vi "Lab Panel V5.28.vi"() -> ()   [LabVIEW 2013] (continued)
              tunnel: w5214 -> [_ w5263]
              tunnel: w5224 -> [_ w5262]
              tunnel: w5223 -> [_ w5261]
              tunnel: w5222 -> [_ w5260]
              tunnel: w5221 -> [_ w5259]
              tunnel: w5220 -> [_ w5258]
              tunnel: w5219 -> [_ w5257]
              tunnel: w5218 -> [_ w5256]
              tunnel: w5217 -> [_ w5255]
              tunnel: w5216 -> [_ w5254]
              tunnel: w5215 -> [_ w5253]
              tunnel: "TO (string):" -> [w5229 _]
              frame #0 {
                # "mail test"
                n2896 = case shown="True" w5230 {
                  tunnel: w5233 -> [_ w5237]
                  tunnel: w5229 -> [_ w5236]
                  tunnel: w5232 -> [_ w5235]
                  tunnel: w5231 -> [_ w5234]
                  frame False {
                  }
                  frame True {
                    n2897 = stacked-sequence {
                      seq-local: [_ _ w5247 _] -> [_ _ _ w5248]
                      tunnel: w5237 -> [w5240 _ _ w5252]
                      tunnel: w5236 -> [_ _ w5245 _]
                      tunnel: w5235 -> [_ _ w5243 _]
                      tunnel: w5234 -> [_ _ w5244 _]
                      frame #0 {
                        n2898 = Bundle(cluster=w5240, "TEST MAIL STATUS"="TEST START") -> (w5238:T7)  [unwired: 6 in]
                        n2899 = local write "MAIL SETTINGS"(w5238) -> ()
                      }
                      frame #1 {
                        n2900 = Wait (ms)(milliseconds to wait=500) -> ()  [unwired: 1 out]
                      }
                      frame #2 {
                        n2901 = call "sub vi - send mail v5.vi"("TO:"=w5245, "subject"="MAIL TEST FROM LAB PANEL", "from"=w5244, "out going server"=w5243, "message"="TEST MESSAGE") -> ("error out"=w5247:errorcluster)  [unwired: 10 in]
                      }
                      frame #3 {
                        n2902 = Bundle(cluster=w5252, "TEST MAIL"=FALSE, "TEST MAIL STATUS"="TEST END", "mail error"=w5248) -> (w5250:T7)  [unwired: 4 in]
                        n2903 = local write "MAIL SETTINGS"(w5250) -> ()
                      }
                    }
                  }
                }
              }
              frame #1 {
                # "mail report"
                n2904 = stacked-sequence {
                  seq-local: [_ w5310 _ _] -> [_ _ _ w5500]
                  seq-local: [_ _ w5413 _] -> [_ _ _ w5490]
                  seq-local: [w5277 _ _ _] -> [_ w5327 _ _]
                  seq-local: [w5276 _ _ _] -> [_ w5326 _ _]
                  seq-local: [w5274 _ _ _] -> [_ w5324 _ _]
                  seq-local: [w5275 _ _ _] -> [_ w5325 _ _]
                  seq-local: [w5273 _ _ _] -> [_ w5323 _ _]
                  seq-local: [w5272 _ _ _] -> [_ w5318 _ _]
                  seq-local: [w5271 _ _ _] -> [_ w5319 _ _]
                  seq-local: [w5270 _ _ _] -> [_ w5320 _ _]
                  seq-local: [w5269 _ _ _] -> [_ w5321 _ _]
                  seq-local: [w5268 _ _ _] -> [_ w5322 _ _]
                  tunnel: w5267 -> [_ _ _ w5501]
                  tunnel: w5266 -> [_ _ _ w5484]
                  tunnel: w5265 -> [_ _ _ w5498]
                  tunnel: w5264 -> [_ _ _ w5497]
                  tunnel: w5263 -> [w5308 _ _ w5492]
                  tunnel: w5262 -> [_ _ w5443 _]
                  tunnel: w5261 -> [_ _ w5440 _]
                  tunnel: w5260 -> [_ _ w5439 _]
                  tunnel: w5259 -> [_ _ w5438 _]
                  tunnel: w5258 -> [_ _ w5437 _]
                  tunnel: w5257 -> [_ _ w5436 _]
                  tunnel: w5256 -> [_ _ w5435 _]
                  tunnel: w5255 -> [_ _ w5434 _]
                  tunnel: w5254 -> [_ _ w5433 _]
                  tunnel: w5253 -> [_ _ w5432 _]
                  frame #0 {
                    n2905 = case shown="False" w5308 {
                      frame False {
                        n2906 = local write "mail control"("") -> ()
                      }
                      frame True {
                      }
                    }
                    n2907 = local read "SET LAB01-1"() -> (w5307:T5)
                    n2908 = local read "SET LAB01-2"() -> (w5306:T5)
                    n2909 = local read "SET LAB02-1"() -> (w5305:T5)
                    n2910 = local read "SET LAB02-2"() -> (w5304:T5)
                    n2911 = local read "SET LAB03-1"() -> (w5303:T5)
                    n2912 = local read "SET LAB04-1"() -> (w5301:T5)
                    n2913 = local read "SET LAB05-1"() -> (w5299:T5)
                    n2914 = local read "SET LAB03-2"() -> (w5302:T5)
                    n2915 = local read "SET LAB04-2"() -> (w5300:T5)
                    n2916 = local read "SET LAB05-2"() -> (w5298:T5)
                    n2917 = Unbundle(w5303) -> ("DESCRIPTION"=w5283:string)  [unwired: 4 out]
                    n2918 = Unbundle(w5302) -> ("DESCRIPTION"=w5282:string)  [unwired: 4 out]
                    n2919 = Unbundle(w5301) -> ("DESCRIPTION"=w5281:string)  [unwired: 4 out]
                    n2920 = Unbundle(w5298) -> ("DESCRIPTION"=w5278:string)  [unwired: 4 out]
                    n2921 = Unbundle(w5304) -> ("DESCRIPTION"=w5284:string)  [unwired: 4 out]
                    n2922 = Unbundle(w5300) -> ("DESCRIPTION"=w5280:string)  [unwired: 4 out]
                    n2923 = Unbundle(w5307) -> ("DESCRIPTION"=w5296:string)  [unwired: 4 out]
                    n2924 = Unbundle(w5305) -> ("DESCRIPTION"=w5285:string)  [unwired: 4 out]
                    n2925 = Unbundle(w5299) -> ("DESCRIPTION"=w5279:string)  [unwired: 4 out]
                    n2926 = Unbundle(w5306) -> ("DESCRIPTION"=w5286:string)  [unwired: 4 out]
                    n2927 = Concatenate Strings("[LAB05-2/", w5278) -> (w5268:string)
                    n2928 = Concatenate Strings("[LAB05-1/", w5279) -> (w5269:string)
                    n2929 = Concatenate Strings("[LAB04-2/", w5280) -> (w5270:string)
                    n2930 = Concatenate Strings("[LAB03-2/", w5282) -> (w5272:string)
                    n2931 = Concatenate Strings("[LAB04-1/", w5281) -> (w5271:string)
                    n2932 = Concatenate Strings("[LAB03-1/", w5283) -> (w5273:string)
                    n2933 = Concatenate Strings("[LAB01-2/", w5286) -> (w5276:string)
                    n2934 = Concatenate Strings("[LAB02-2/", w5284) -> (w5274:string)
                    n2935 = Concatenate Strings("[LAB01-1/", w5296) -> (w5277:string)
                    n2936 = Concatenate Strings("[LAB02-1/", w5285) -> (w5275:string)
                  }
                  frame #1 {
                    w5331 = "/"
                    w5332 = 2.0
                    n2937 = local read "DISP LAB01-2"() -> (w5411:T4)
                    n2938 = local read "DISP LAB01-1"() -> (w5412:T4)
                    n2939 = local read "DISP LAB02-1"() -> (w5410:T4)
                    n2940 = local read "DISP LAB03-2"() -> (w5407:T4)
                    n2941 = local read "DISP LAB02-2"() -> (w5409:T4)
                    n2942 = local read "DISP LAB03-1"() -> (w5408:T4)
                    n2943 = local read "DISP LAB04-2"() -> (w5405:T4)
                    n2944 = local read "DISP LAB04-1"() -> (w5406:T4)
                    n2945 = local read "DISP LAB05-1"() -> (w5404:T4)
                    n2946 = local read "DISP LAB05-2"() -> (w5403:T4)
                    n2947 = Unbundle(w5411) -> ("CYCLE"=w5395:dbl, "MINS"=w5394:dbl, "STATUS"=w5391:string)
                    n2948 = Unbundle(w5412) -> ("CYCLE"=w5400:dbl, "MINS"=w5399:dbl, "STATUS"=w5396:string)
                    n2949 = Unbundle(w5410) -> ("CYCLE"=w5388:dbl, "MINS"=w5387:dbl, "STATUS"=w5386:string)
                    n2950 = Unbundle(w5407) -> ("CYCLE"=w5375:dbl, "MINS"=w5374:dbl, "STATUS"=w5371:string)
                    n2951 = Unbundle(w5408) -> ("CYCLE"=w5380:dbl, "MINS"=w5379:dbl, "STATUS"=w5376:string)
                    n2952 = Unbundle(w5409) -> ("CYCLE"=w5385:dbl, "MINS"=w5384:dbl, "STATUS"=w5381:string)
                    n2953 = Unbundle(w5406) -> ("CYCLE"=w5370:dbl, "MINS"=w5369:dbl, "STATUS"=w5366:string)
                    n2954 = Unbundle(w5405) -> ("CYCLE"=w5365:dbl, "MINS"=w5364:dbl, "STATUS"=w5361:string)
                    n2955 = Unbundle(w5404) -> ("CYCLE"=w5360:dbl, "MINS"=w5359:dbl, "STATUS"=w5356:string)
                    n2956 = Unbundle(w5403) -> ("CYCLE"=w5402:dbl, "MINS"=w5401:dbl, "STATUS"=w5353:string)
                    n2957 = Number To Decimal String(number=w5388) -> (decimal integer string=w5390:string)  [unwired: 1 in]
                    n2958 = Number To Decimal String(number=w5385) -> (decimal integer string=w5383:string)  [unwired: 1 in]
                    n2959 = Number To Decimal String(number=w5380) -> (decimal integer string=w5378:string)  [unwired: 1 in]
                    n2960 = Number To Decimal String(number=w5395) -> (decimal integer string=w5393:string)  [unwired: 1 in]
                    n2961 = Number To Decimal String(number=w5375) -> (decimal integer string=w5373:string)  [unwired: 1 in]
                    n2962 = Number To Decimal String(number=w5400) -> (decimal integer string=w5398:string)  [unwired: 1 in]
                    n2963 = Number To Decimal String(number=w5402) -> (decimal integer string=w5355:string)  [unwired: 1 in]
                    n2964 = Number To Decimal String(number=w5370) -> (decimal integer string=w5368:string)  [unwired: 1 in]
                    n2965 = Number To Decimal String(number=w5365) -> (decimal integer string=w5363:string)  [unwired: 1 in]
                    n2966 = Number To Decimal String(number=w5360) -> (decimal integer string=w5358:string)  [unwired: 1 in]
                    n2967 = Number To Fractional String(number=w5387, precision (6)=w5332) -> (F-format string=w5389:string)  [unwired: 2 in]
                    n2968 = Number To Fractional String(number=w5374, precision (6)=w5332) -> (F-format string=w5372:string)  [unwired: 2 in]
                    n2969 = Number To Fractional String(number=w5384, precision (6)=w5332) -> (F-format string=w5382:string)  [unwired: 2 in]
                    n2970 = Number To Fractional String(number=w5379, precision (6)=w5332) -> (F-format string=w5377:string)  [unwired: 2 in]
                    n2971 = Number To Fractional String(number=w5364, precision (6)=w5332) -> (F-format string=w5362:string)  [unwired: 2 in]
                    n2972 = Number To Fractional String(number=w5369, precision (6)=w5332) -> (F-format string=w5367:string)  [unwired: 2 in]
                    n2973 = Number To Fractional String(number=w5394, precision (6)=w5332) -> (F-format string=w5392:string)  [unwired: 2 in]
                    n2974 = Number To Fractional String(number=w5359, precision (6)=w5332) -> (F-format string=w5357:string)  [unwired: 2 in]
                    n2975 = Number To Fractional String(number=w5399, precision (6)=w5332) -> (F-format string=w5397:string)  [unwired: 2 in]
                    n2976 = Number To Fractional String(number=w5401, precision (6)=w5332) -> (F-format string=w5354:string)  [unwired: 2 in]
                    n2977 = Concatenate Strings(w5331, w5373, w5331, w5372, w5331, w5371) -> (w5347:string)
                    n2978 = Concatenate Strings(w5331, w5368, w5331, w5367, w5331, w5366) -> (w5346:string)
                    n2979 = Concatenate Strings(w5331, w5363, w5331, w5362, w5331, w5361) -> (w5345:string)
                    n2980 = Concatenate Strings(w5331, w5358, w5331, w5357, w5331, w5356) -> (w5344:string)
                    n2981 = Concatenate Strings(w5331, w5355, w5331, w5354, w5331, w5353) -> (w5343:string)
                    n2982 = Concatenate Strings(w5331, w5398, w5331, w5397, w5331, w5396) -> (w5352:string)
                    n2983 = Concatenate Strings(w5331, w5378, w5331, w5377, w5331, w5376) -> (w5348:string)
                    n2984 = Concatenate Strings(w5331, w5393, w5331, w5392, w5331, w5391) -> (w5351:string)
                    n2985 = Concatenate Strings(w5331, w5390, w5331, w5389, w5331, w5386) -> (w5350:string)
                    n2986 = Concatenate Strings(w5331, w5383, w5331, w5382, w5331, w5381) -> (w5349:string)
                    n2987 = Concatenate Strings("]", "\r") -> (w5328:string)
                    n2988 = Concatenate Strings(w5323, w5348, w5328) -> (w5338:string)
                    n2989 = Concatenate Strings(w5325, w5350, w5328) -> (w5340:string)
                    n2990 = Concatenate Strings(w5324, w5349, w5328) -> (w5339:string)
                    n2991 = Concatenate Strings(w5320, w5345, w5328) -> (w5335:string)
                    n2992 = Concatenate Strings(w5321, w5344, w5328) -> (w5336:string)
                    n2993 = Concatenate Strings(w5319, w5346, w5328) -> (w5334:string)
                    n2994 = Concatenate Strings(w5318, w5347, w5328) -> (w5333:string)
                    n2995 = Concatenate Strings(w5322, w5343, w5328) -> (w5337:string)
                    n2996 = Concatenate Strings(w5326, w5351, w5328) -> (w5341:string)
                    n2997 = Concatenate Strings(w5327, w5352, w5328) -> (w5342:string)
                    n2998 = Concatenate Strings(w5342, w5341, w5340, w5339, w5338, w5333, w5334, w5335, w5336, w5337) -> (w5311:string)
                    n2999 = Concatenate Strings("[PANEL/", "DESC/", "CYCLES/", "MINS/", "STATUS]", "\r", w5311) -> (w5310:string)
                    "MAIL REPORT" <- w5310
                    n3000 = global write "Global display 3.vi" "log all"(w5310) -> ()
                  }
                  frame #2 {
                    w5441 = "END"
                    n3001 = local read "mail control"() -> (w5442:string)
                    n3002 = case shown="False" w5437 {
                      tunnel: w5442 -> [w5466 _]
                      tunnel: w5441 -> [w5465 _]
                      tunnel: [w5464 FALSE] -> w5427
                      frame False {
                        n3003 = Equal?(x=w5466, y=w5465) -> (x = y?=w5464:bool)
                      }
                      frame True {
                      }
                    }
                    n3004 = case shown="False" w5443 {
                      tunnel: w5442 -> [w5482 _]
                      tunnel: w5441 -> [w5481 _]
                      tunnel: [w5480 FALSE] -> w5431
                      frame False {
                        n3005 = Equal?(x=w5482, y=w5481) -> (x = y?=w5480:bool)
                      }
                      frame True {
                      }
                    }
                    n3006 = case shown="False" w5440 {
                      tunnel: w5442 -> [w5478 _]
                      tunnel: w5441 -> [w5477 _]
                      tunnel: [w5476 FALSE] -> w5430
                      frame False {
                        n3007 = Equal?(x=w5478, y=w5477) -> (x = y?=w5476:bool)
                      }
                      frame True {
                      }
                    }
                    n3008 = case shown="False" w5438 {
                      tunnel: w5442 -> [w5470 _]
                      tunnel: w5441 -> [w5469 _]
                      tunnel: [w5468 FALSE] -> w5428
                      frame False {
                        n3009 = Equal?(x=w5470, y=w5469) -> (x = y?=w5468:bool)
                      }
                      frame True {
                      }
                    }
                    n3010 = case shown="False" w5439 {
                      tunnel: w5442 -> [w5474 _]
                      tunnel: w5441 -> [w5473 _]
                      tunnel: [w5472 FALSE] -> w5429
                      frame False {
                        n3011 = Equal?(x=w5474, y=w5473) -> (x = y?=w5472:bool)
                      }
                      frame True {
                      }
                    }
                    n3012 = Or(x=w5429, y=w5428) -> (x .or. y?=w5420:bool)
                    n3013 = Or(x=w5431, y=w5430) -> (x .or. y?=w5421:bool)
                    n3014 = Or(x=w5421, y=w5420) -> (x .or. y?=w5416:bool)
                    n3015 = case shown="False" w5433 {
                      tunnel: w5442 -> [w5450 _]
                      tunnel: w5441 -> [w5449 _]
                      tunnel: [w5448 FALSE] -> w5422
                      frame False {
                        n3016 = Equal?(x=w5450, y=w5449) -> (x = y?=w5448:bool)
                      }
                      frame True {
                      }
                    }
                    n3017 = case shown="False" w5432 {
                      tunnel: w5442 -> [w5446 _]
                      tunnel: w5441 -> [w5445 _]
                      tunnel: [w5444 FALSE] -> w5426
                      frame False {
                        n3018 = Equal?(x=w5446, y=w5445) -> (x = y?=w5444:bool)
                      }
                      frame True {
                      }
                    }
                    n3019 = case shown="False" w5434 {
                      tunnel: w5442 -> [w5454 _]
                      tunnel: w5441 -> [w5453 _]
                      tunnel: [w5452 FALSE] -> w5423
                      frame False {
                        n3020 = Equal?(x=w5454, y=w5453) -> (x = y?=w5452:bool)
                      }
                      frame True {
                      }
                    }
                    n3021 = case shown="False" w5436 {
                      tunnel: w5442 -> [w5462 _]
                      tunnel: w5441 -> [w5461 _]
                      tunnel: [w5460 FALSE] -> w5425
                      frame False {
                        n3022 = Equal?(x=w5462, y=w5461) -> (x = y?=w5460:bool)
                      }
                      frame True {
                      }
                    }
                    n3023 = case shown="False" w5435 {
                      tunnel: w5442 -> [w5458 _]
                      tunnel: w5441 -> [w5457 _]
                      tunnel: [w5456 FALSE] -> w5424
                      frame False {
                        n3024 = Equal?(x=w5458, y=w5457) -> (x = y?=w5456:bool)
                      }
                      frame True {
                      }
                    }
                    n3025 = Or(x=w5425, y=w5424) -> (x .or. y?=w5419:bool)
                    n3026 = Or(x=w5423, y=w5422) -> (x .or. y?=w5418:bool)
                    n3027 = Or(x=w5426, y=w5427) -> (x .or. y?=w5414:bool)
                    n3028 = Or(x=w5419, y=w5418) -> (x .or. y?=w5417:bool)
                    n3029 = Or(x=w5416, y=w5417) -> (x .or. y?=w5415:bool)
                    n3030 = Or(x=w5415, y=w5414) -> (x .or. y?=w5413:bool)
                  }
                  frame #3 {
                    n3031 = local read "on loops"() -> (w5496:dbl)
                    n3032 = local read "jig cycle"() -> (w5493:dbl)
                    n3033 = local read "Send Mail Now"() -> (w5487:bool)
                    n3034 = Add(x=w5496, y=5.0) -> (x+y=w5494:dbl)
                    n3035 = Equal?(x=w5493, y=w5494) -> (x = y?=w5488:bool)
                    n3036 = And(x=w5488, y=w5487) -> (x .and. y?=w5486:bool)
                    n3037 = And(x=w5492, y=w5488) -> (x .and. y?=w5491:bool)
                    n3038 = And(x=w5491, y=w5490) -> (x .and. y?=w5489:bool)
                    n3039 = Or(x=w5489, y=w5486) -> (x .or. y?=w5485:bool)
                    n3040 = case shown="True" w5485 {
                      tunnel: w5501 -> [_ w5507]
                      tunnel: w5500 -> [_ w5506]
                      tunnel: "Lab Panel Test Status" -> [_ w5505]
                      tunnel: w5498 -> [_ w5504]
                      tunnel: w5497 -> [_ w5503]
                      tunnel: w5484 -> [_ w5502]
                      frame False {
                      }
                      frame True {
                        n3041 = stacked-sequence {
                          tunnel: w5507 -> [w5516 _]
                          tunnel: w5506 -> [w5515 _]
                          tunnel: w5505 -> [w5514 _]
                          tunnel: w5504 -> [w5513 _]
                          tunnel: w5503 -> [w5512 _]
                          tunnel: w5502 -> [w5511 _]
                          frame #0 {
                            n3042 = call "sub vi - send mail v5.vi"("TO:"=w5516, "subject"=w5514, "Info"="Test station status report", "from"=w5512, "out going server"=w5513, "message"=w5515) -> ("error out"=w5510:errorcluster)  [unwired: 9 in]
                            n3043 = Bundle(cluster=w5511, "mail error"=w5510) -> (w5509:T7)  [unwired: 6 in]
                            n3044 = local write "MAIL SETTINGS"(w5509) -> ()
                          }
                          frame #1 {
                            n3045 = local write "mail control"("") -> ()
                            n3046 = local write "Send Mail Now"(FALSE) -> ()
                          }
                        }
                      }
                    }
                  }
                }
              }
            }
          }
          frame #20 {
            # "save jig cycle values once all run switches are off"
            n3047 = stacked-sequence {
              tunnel: w5528 -> [_ w5557]
              tunnel: w5527 -> [_ w5556]
              tunnel: w5526 -> [_ w5555]
              tunnel: w5525 -> [_ w5554]
              tunnel: w5524 -> [_ w5553]
              tunnel: w5523 -> [_ w5552]
              tunnel: w5522 -> [_ w5551]
              tunnel: w5521 -> [_ w5550]
              tunnel: w5520 -> [_ w5549]
              tunnel: w5519 -> [_ w5548]
              frame #0 {
              }
              frame #1 {
                n3048 = Not(x=w5548) -> (.not. x?=w5531:bool)
                n3049 = Not(x=w5556) -> (.not. x?=w5546:bool)
                n3050 = Not(x=w5553) -> (.not. x?=w5541:bool)
                n3051 = Not(x=w5551) -> (.not. x?=w5537:bool)
                n3052 = Not(x=w5549) -> (.not. x?=w5533:bool)
                n3053 = Not(x=w5557) -> (.not. x?=w5547:bool)
                n3054 = Not(x=w5555) -> (.not. x?=w5545:bool)
                n3055 = Not(x=w5552) -> (.not. x?=w5539:bool)
                n3056 = Not(x=w5554) -> (.not. x?=w5543:bool)
                n3057 = Not(x=w5550) -> (.not. x?=w5535:bool)
                n3058 = local read "Save JC"() -> (w5559:bool)
                n3059 = And(x=w5547, y=w5546) -> (x .and. y?=w5544:bool)
                n3060 = And(x=w5544, y=w5545) -> (x .and. y?=w5542:bool)
                n3061 = And(x=w5542, y=w5543) -> (x .and. y?=w5540:bool)
                n3062 = And(x=w5540, y=w5541) -> (x .and. y?=w5538:bool)
                n3063 = And(x=w5538, y=w5539) -> (x .and. y?=w5536:bool)
                n3064 = And(x=w5536, y=w5537) -> (x .and. y?=w5534:bool)
                n3065 = And(x=w5534, y=w5535) -> (x .and. y?=w5532:bool)
                n3066 = And(x=w5532, y=w5533) -> (x .and. y?=w5530:bool)
                n3067 = And(x=w5530, y=w5531) -> (x .and. y?=w5529:bool)
                n3068 = And(x=w5529, y=w5559) -> (x .and. y?=w5558:bool)
                n3069 = case shown="True" w5558 {
                  tunnel: w5529 -> [w5560 _]
                  frame False {
                    n3070 = case shown="False" w5560 {
                      frame False {
                        n3071 = local write "Save JC"(TRUE) -> ()
                      }
                      frame True {
                      }
                    }
                  }
                  frame True {
                    n3072 = stacked-sequence {
                      frame #0 {
                        n3073 = String To Path(string="c:\\crabtree\\Jig Cycles\\") -> (path=w5572:path)
                        n3074 = Build Path(base path=w5572, name or relative path="jigcycles.bin") -> (appended path=w5570:path)
                        n3075 = Create Folder(path (use dialog)=w5572) -> (error out=w5574:errorcluster)  [unwired: 2 in, 2 out]
                        n3076 = local read "JIG RELAY CYCLES"() -> (w5564:T8)
                        n3077 = call <vilib>:"Clear Errors.vi"("error in (no error)"=w5574) -> ()  [unwired: 6 in, 1 out]
                        n3078 = local write "Save JC"(FALSE) -> ()
                        n3079 = Open/Create/Replace File(file path (use dialog)=w5570, operation (0:open)=T17."replace or create") -> (refnum out=w5568:refnum<file>, error out=w5569:errorcluster)  [unwired: 4 in, 1 out]
                        n3080 = Write to Binary File(file (use dialog)=w5568, data=w5564, error in=w5569) -> (refnum out=w5567:refnum<file>, error out=w5566:errorcluster)  [unwired: 3 in, 1 out]
                        n3081 = Close File(refnum=w5567, error in=w5566) -> (error out=w5565:errorcluster)  [unwired: 1 out]
                        n3082 = local write "data file error"(w5565) -> ()
                      }
                      frame #1 {
                        n3083 = local read "JIG RELAY CYCLES"() -> (w5597:T8)
                        n3084 = Unbundle By Name(w5597) -> ("LAB01-1"=w5592:dbl, "LAB01-2"=w5591:dbl, "LAB02-1"=w5589:dbl, "LAB02-2"=w5588:dbl, "LAB03-1"=w5586:dbl, "LAB03-2"=w5583:dbl, "LAB04-1"=w5582:dbl, "LAB04-2"=w5580:dbl, "LAB05-1"=w5578:dbl, "LAB05-2"=w5576:dbl)
                        n3085 = stacked-sequence {
                          tunnel: w5592 -> [w5600 _ _ _ _ _ _ _ _ _]
                          tunnel: 1000000 -> [w5603 w5613 w5623 w5633 w5643 w5653 w5663 w5673 w5683 w5693]
                          tunnel: [w5601 _ _ _ _ _ _ _ _ _] -> w5595
                          tunnel: "TEST STATION HAS REACHED 1 MILLION CYCLES, REPLACE  CONTROL RELAYS" -> [w5599 w5611 w5621 w5631 w5641 w5651 w5661 w5671 w5681 w5691]
                          tunnel: [_ w5610 _ _ _ _ _ _ _ _] -> w5593
                          tunnel: w5591 -> [_ w5609 _ _ _ _ _ _ _ _]
                          tunnel: [_ _ w5620 _ _ _ _ _ _ _] -> w5590
                          tunnel: w5589 -> [_ _ w5619 _ _ _ _ _ _ _]
                          tunnel: w5588 -> [_ _ _ w5630 _ _ _ _ _ _]
                          tunnel: [_ _ _ w5629 _ _ _ _ _ _] -> w5587
                          tunnel: w5586 -> [_ _ _ _ w5640 _ _ _ _ _]
                          tunnel: [_ _ _ _ w5639 _ _ _ _ _] -> w5585
                          tunnel: [_ _ _ _ _ w5650 _ _ _ _] -> w5584
                          tunnel: w5583 -> [_ _ _ _ _ w5649 _ _ _ _]
                          tunnel: w5582 -> [_ _ _ _ _ _ w5660 _ _ _]
                          tunnel: [_ _ _ _ _ _ w5659 _ _ _] -> w5581
                          tunnel: w5580 -> [_ _ _ _ _ _ _ w5670 _ _]
                          tunnel: [_ _ _ _ _ _ _ w5669 _ _] -> w5579
                          tunnel: w5578 -> [_ _ _ _ _ _ _ _ w5680 _]
                          tunnel: [_ _ _ _ _ _ _ _ w5679 _] -> w5577
                          tunnel: w5576 -> [_ _ _ _ _ _ _ _ _ w5690]
                          tunnel: [_ _ _ _ _ _ _ _ _ w5689] -> w5575
                          frame #0 {
                            n3086 = Greater?(x=w5600, y=w5603) -> (0:w5602:bool)
                            n3087 = case shown="True" w5602 {
                              tunnel: [w5604 0] -> w5601
                              tunnel: w5600 -> [w5604 _]
                              tunnel: w5599 -> [_ w5605]
                              frame False {
                              }
                              frame True {
                                n3088 = Concatenate Strings("LA01-1 ", w5605) -> (w5608:string)
                                n3089 = One Button Dialog(message=w5608) -> ()  [unwired: 1 in, 1 out]
                              }
                            }
                          }
                          frame #1 {
                            n3090 = Greater?(x=w5609, y=w5613) -> (0:w5612:bool)
                            n3091 = case shown="True" w5612 {
                              tunnel: [w5614 0] -> w5610
                              tunnel: w5609 -> [w5614 _]
                              tunnel: w5611 -> [_ w5615]
                              frame False {
                              }
                              frame True {
                                n3092 = Concatenate Strings("LA01-2 ", w5615) -> (w5618:string)
                                n3093 = One Button Dialog(message=w5618) -> ()  [unwired: 1 in, 1 out]
                              }
                            }
                          }
                          frame #2 {
                            n3094 = Greater?(x=w5619, y=w5623) -> (0:w5622:bool)
                            n3095 = case shown="True" w5622 {
                              tunnel: [w5624 0] -> w5620
                              tunnel: w5619 -> [w5624 _]
                              tunnel: w5621 -> [_ w5625]
                              frame False {
                              }
                              frame True {
                                n3096 = Concatenate Strings("LA02-1 ", w5625) -> (w5628:string)
                                n3097 = One Button Dialog(message=w5628) -> ()  [unwired: 1 in, 1 out]
                              }
                            }
                          }
                          frame #3 {
                            n3098 = Greater?(x=w5630, y=w5633) -> (0:w5632:bool)
                            n3099 = case shown="True" w5632 {
                              tunnel: [w5634 0] -> w5629
                              tunnel: w5630 -> [w5634 _]
                              tunnel: w5631 -> [_ w5635]
                              frame False {
                              }
                              frame True {
                                n3100 = Concatenate Strings("LA02-2 ", w5635) -> (w5638:string)
                                n3101 = One Button Dialog(message=w5638) -> ()  [unwired: 1 in, 1 out]
                              }
                            }
                          }
                          frame #4 {
                            n3102 = Greater?(x=w5640, y=w5643) -> (0:w5642:bool)
                            n3103 = case shown="True" w5642 {
                              tunnel: [w5644 0] -> w5639
                              tunnel: w5640 -> [w5644 _]
                              tunnel: w5641 -> [_ w5645]
                              frame False {
                              }
                              frame True {
                                n3104 = Concatenate Strings("LA03-1 ", w5645) -> (w5648:string)
                                n3105 = One Button Dialog(message=w5648) -> ()  [unwired: 1 in, 1 out]
                              }
                            }
                          }
                          frame #5 {
                            n3106 = Greater?(x=w5649, y=w5653) -> (0:w5652:bool)
                            n3107 = case shown="True" w5652 {
                              tunnel: [w5654 0] -> w5650
                              tunnel: w5649 -> [w5654 _]
                              tunnel: w5651 -> [_ w5655]
                              frame False {
                              }
                              frame True {
                                n3108 = Concatenate Strings("LA03-2 ", w5655) -> (w5658:string)
                                n3109 = One Button Dialog(message=w5658) -> ()  [unwired: 1 in, 1 out]
                              }
                            }
                          }
                          frame #6 {
                            n3110 = Greater?(x=w5660, y=w5663) -> (0:w5662:bool)
                            n3111 = case shown="True" w5662 {
                              tunnel: [w5664 0] -> w5659
                              tunnel: w5660 -> [w5664 _]
                              tunnel: w5661 -> [_ w5665]
                              frame False {
                              }
                              frame True {
                                n3112 = Concatenate Strings("LA04-1 ", w5665) -> (w5668:string)
                                n3113 = One Button Dialog(message=w5668) -> ()  [unwired: 1 in, 1 out]
                              }
                            }
                          }
                          frame #7 {
                            n3114 = Greater?(x=w5670, y=w5673) -> (0:w5672:bool)
                            n3115 = case shown="True" w5672 {
                              tunnel: [w5674 0] -> w5669
                              tunnel: w5670 -> [w5674 _]
                              tunnel: w5671 -> [_ w5675]
                              frame False {
                              }
                              frame True {
                                n3116 = Concatenate Strings("LA04-2 ", w5675) -> (w5678:string)
                                n3117 = One Button Dialog(message=w5678) -> ()  [unwired: 1 in, 1 out]
                              }
                            }
                          }
                          frame #8 {
                            n3118 = Greater?(x=w5680, y=w5683) -> (0:w5682:bool)
                            n3119 = case shown="True" w5682 {
                              tunnel: [w5684 0] -> w5679
                              tunnel: w5680 -> [w5684 _]
                              tunnel: w5681 -> [_ w5685]
                              frame False {
                              }
                              frame True {
                                n3120 = Concatenate Strings("LA05-1 ", w5685) -> (w5688:string)
                                n3121 = One Button Dialog(message=w5688) -> ()  [unwired: 1 in, 1 out]
                              }
                            }
                          }
                          frame #9 {
                            n3122 = Greater?(x=w5690, y=w5693) -> (0:w5692:bool)
                            n3123 = case shown="True" w5692 {
                              tunnel: [w5694 0] -> w5689
                              tunnel: w5690 -> [w5694 _]
                              tunnel: w5691 -> [_ w5695]
                              frame False {
                              }
                              frame True {
                                n3124 = Concatenate Strings("LA05-2 ", w5695) -> (w5698:string)
                                n3125 = One Button Dialog(message=w5698) -> ()  [unwired: 1 in, 1 out]
                              }
                            }
                          }
                        }
                        n3126 = Bundle By Name(cluster=w5597, "LAB01-1"=w5595, "LAB01-2"=w5593, "LAB02-1"=w5590, "LAB02-2"=w5587, "LAB03-1"=w5585, "LAB03-2"=w5584, "LAB04-1"=w5581, "LAB04-2"=w5579, "LAB05-1"=w5577, "LAB05-2"=w5575) -> (w5596:T8)
                        n3127 = local write "JIG RELAY CYCLES"(w5596) -> ()
                      }
                    }
                  }
                }
              }
            }
          }
          frame #21 {
            # "get temperature values"
            n3128 = local read "Simulate"() -> (w5711:bool)
            n3129 = local read "Temp Test Cal"() -> (w5708:dbl)
            n3130 = stacked-sequence {
              seq-local: [w5713 _] -> [_ w5758]
              tunnel: w5711 -> [_ w5771]
              tunnel: T14 {"1  (A) cal"=1.0, "1 (V) cal"=1.0, "1 (PF) cal"=1.0, "1 (TL) cal"=1.0, "1 (TN) cal"=1.0, "2 (A) cal"=1.0, "2 (V) cal"=1.0, "2 (PF) cal"=1.0, "2 (TL) cal"=1.0, "2 (TN) cal"=1.0} ("CAL LAB01") -> [_ w5770]
              tunnel: w5709 -> [_ w5769]
              tunnel: w5708 -> [_ w5768]
              tunnel: w5707 -> [_ w5767]
              tunnel: w5706 -> [_ w5766]
              tunnel: w5705 -> [_ w5765]
              tunnel: w5704 -> [_ w5764]
              tunnel: w5703 -> [_ w5763]
              tunnel: w5702 -> [_ w5762]
              tunnel: w5701 -> [_ w5761]
              tunnel: w5700 -> [_ w5760]
              tunnel: w5699 -> [_ w5759]
              frame #0 {
                # "only get temperature from initial valid temperature circuits"
                n3131 = local read "Select COM port"() -> (w5721:refnum<visa-resource-name>)
                "COM port" <- w5721
                n3132 = global write "Global 1.vi" "COM port"(w5721) -> ()
                n3133 = local read "Temp read loop"() -> (w5718:dbl)
                n3134 = global write "Global 1.vi" "tmp dly lps"("Temp Delay Lps") -> ()
                n3135 = global write "Global 1.vi" "dly value"("Temp Value") -> ()
                n3136 = local read "jig cycle"() -> (w5722:dbl)
                n3137 = local read "on loops"() -> (w5724:dbl)
                n3138 = Equal?(x=w5718, y=1) -> (x = y?=w5715:bool)
                n3139 = Add(x=w5724, y=6) -> (x+y=w5725:dbl)
                n3140 = Equal?(x=w5722, y=w5725) -> (x = y?=w5716:bool)
                n3141 = And(x=w5716, y=w5715) -> (x .and. y?=w5714:bool)
                n3142 = Or(x=w5714, y="Read Temp") -> (x .or. y?=w5713:bool)
                n3143 = case shown="True" w5713 {
                  frame False {
                  }
                  frame True {
                    n3144 = local read "Simulate"() -> (w5727:bool)
                    n3145 = local write "TEMP"(TRUE) -> ()
                    n3146 = local write "Read Temp"(FALSE) -> ()
                    n3147 = stacked-sequence {
                      tunnel: 1.0 -> [_ _ _ _ w5757]
                      tunnel: w5727 -> [_ _ _ _ w5756]
                      frame #0 {
                        # "only switch relay on to reset temp circuits if busy testing"
                        n3148 = disable-structure shown="Disabled" {
                          frame Disabled {
                            n3149 = local read "Any Test Running"() -> ()  [unwired: 1 out]
                          }
                          frame Enabled {
                          }
                        }
                        n3150 = local read "USB OUT 0"() -> (w5731:bool[])
                        n3151 = local read "USB OUT 2"() -> (w5733:bool[])
                        n3152 = local read "USB OUT 1"() -> (w5732:bool[])
                        n3153 = Insert Into Array(array=w5733, index=7, new element=TRUE) -> (w5734:bool[])
                        n3154 = call "sub vi - Drive Relays All v6.vi"("Array #2"=w5734, "Array #1"=w5732, "Array #0"=w5731) -> ()  [unwired: 8 in, 1 out]
                      }
                      frame #1 {
                        # "time delay"
                        n3155 = Wait (ms)(milliseconds to wait=500) -> ()  [unwired: 1 out]
                      }
                      frame #2 {
                        # "switch relay off"
                        n3156 = local read "USB OUT 0"() -> (w5737:bool[])
                        n3157 = local read "USB OUT 2"() -> (w5739:bool[])
                        n3158 = local read "USB OUT 1"() -> (w5738:bool[])
                        n3159 = Insert Into Array(array=w5739, index=7, new element=FALSE) -> (w5740:bool[])
                        n3160 = call "sub vi - Drive Relays All v6.vi"("Array #2"=w5740, "Array #1"=w5738, "Array #0"=w5737) -> ()  [unwired: 8 in, 1 out]
                      }
                      frame #3 {
                        # "time delay"
                        n3161 = Wait (ms)(milliseconds to wait=300) -> ()  [unwired: 1 out]
                      }
                      frame #4 {
                        # "read all valid temp circuits"
                        n3162 = local read "LAB01-TP"() -> (w5749:bool)
                        n3163 = local read "LAB03-TP"() -> (w5747:bool)
                        n3164 = local read "LAB02-TP"() -> (w5748:bool)
                        n3165 = local read "LAB04-TP"() -> (w5746:bool)
                        n3166 = local read "LAB05-TP"() -> (w5750:bool)
                        n3167 = call "sub vi - GET ALL TEMP v7.vi"("LA01-EN"=w5749, "simulate"=w5756, "LA02-EN"=w5748, "LA03-EN"=w5747, "LA04-EN"=w5746, "LA05-EN"=w5750, "Gen Cal Value"=w5757) -> ("LOOP TIME"=→"Read Time":dbl, "LA01 TEMP"=w5755:T25, "LA02 TEMP"=w5754:T25, "LA03 TEMP"=w5753:T25, "LA04 TEMP"=w5752:T25, "error"=→"Error Temp":bool, "LA05 TEMP"=w5751:T25)  [unwired: 1 in, 1 out]
                        n3168 = local write "LAB01 TEMP"(w5755) -> ()
                        n3169 = local write "LAB02 TEMP"(w5754) -> ()
                        n3170 = local write "LAB03 TEMP"(w5753) -> ()
                        n3171 = local write "LAB04 TEMP"(w5752) -> ()
                        n3172 = local write "LAB05 TEMP"(w5751) -> ()
                      }
                    }
                  }
                }
              }
              frame #1 {
                n3173 = case shown="True" w5758 {
                  tunnel: w5771 -> [_ w5784]
                  tunnel: w5770 -> [_ w5783]
                  tunnel: w5769 -> [_ w5782]
                  tunnel: w5768 -> [_ w5781]
                  tunnel: w5767 -> [_ w5780]
                  tunnel: w5766 -> [_ w5779]
                  tunnel: w5765 -> [_ w5778]
                  tunnel: w5764 -> [_ w5777]
                  tunnel: w5763 -> [_ w5776]
                  tunnel: w5762 -> [_ w5775]
                  tunnel: w5761 -> [_ w5774]
                  tunnel: w5760 -> [_ w5773]
                  tunnel: w5759 -> [_ w5772]
                  frame False {
                  }
                  frame True {
                    n3174 = stacked-sequence {
                      tunnel: w5784 -> [_ w5797 w5842 w5887 w5932 w5977 _]
                      tunnel: w5783 -> [_ w5796 w5841 w5886 w5931 w5976 _]
                      tunnel: w5782 -> [_ w5786 _ _ _ _ _]
                      tunnel: w5781 -> [_ w5791 w5840 w5885 w5930 w5975 _]
                      tunnel: w5780 -> [_ w5785 _ _ _ _ _]
                      tunnel: w5779 -> [_ _ w5831 _ _ _ _]
                      tunnel: w5778 -> [_ _ w5830 _ _ _ _]
                      tunnel: w5777 -> [_ _ _ w5876 _ _ _]
                      tunnel: w5776 -> [_ _ _ w5875 _ _ _]
                      tunnel: w5775 -> [_ _ _ _ w5921 _ _]
                      tunnel: w5774 -> [_ _ _ _ w5920 _ _]
                      tunnel: w5773 -> [_ _ _ _ _ w5966 _]
                      tunnel: w5772 -> [_ _ _ _ _ w5965 _]
                      frame #0 {
                      }
                      frame #1 {
                        n3175 = case shown="False" w5797 {
                          tunnel: [w5828 w5829] -> w5813
                          tunnel: w5796 -> [_ w5829]
                          frame False {
                            n3176 = local read "CAL LAB01"() -> (w5828:T14)
                          }
                          frame True {
                          }
                        }
                        n3177 = local read "TEMP LA01"() -> (w5804:T9)
                        n3178 = local read "LAB01 TEMP"() -> (w5803:T12)
                        n3179 = call "sub vi - temperature delay v4.vi"("2-run"=w5785, "1-run"=w5786, "temp values IN"=w5804, "temp signals"=w5803) -> ("T2-N"=w5799:dbl, "T2-L"=w5800:dbl, "T1-N"=w5801:dbl, "T1-L"=w5802:dbl, "temp values OUT"=w5798:T44)  [unwired: 3 in]
                        n3180 = Unbundle By Name(w5813) -> ("1 (TL) cal"=w5808:dbl, "1 (TN) cal"=w5807:dbl, "2 (TL) cal"=w5806:dbl, "2 (TN) cal"=w5805:dbl)  [unwired: 6 out]
                        n3181 = local write "TEMP LA01"(w5798) -> ()
                        n3182 = Multiply(x=w5802, y=w5808) -> (x*y=w5795:dbl)
                        n3183 = Multiply(x=w5801, y=w5807) -> (x*y=w5793:dbl)
                        n3184 = Multiply(x=w5800, y=w5806) -> (x*y=w5790:dbl)
                        n3185 = Multiply(x=w5799, y=w5805) -> (x*y=w5789:dbl)
                        n3186 = case shown="True" w5786 {
                          tunnel: w5795 -> [w5822 w5827]
                          tunnel: w5791 -> [_ w5825]
                          tunnel: [w5822 w5826] -> w5794
                          tunnel: w5793 -> [w5821 w5824]
                          tunnel: [w5821 w5823] -> w5792
                          frame False {
                          }
                          frame True {
                            n3187 = Multiply(x=w5825, y=w5824) -> (x*y=w5823:dbl)
                            n3188 = Multiply(x=w5825, y=w5827) -> (x*y=w5826:dbl)
                          }
                        }
                        n3189 = case shown="True" w5785 {
                          tunnel: w5790 -> [w5815 w5820]
                          tunnel: w5791 -> [_ w5818]
                          tunnel: [w5815 w5819] -> w5788
                          tunnel: w5789 -> [w5814 w5817]
                          tunnel: [w5814 w5816] -> w5787
                          frame False {
                          }
                          frame True {
                            n3190 = Multiply(x=w5818, y=w5817) -> (x*y=w5816:dbl)
                            n3191 = Multiply(x=w5818, y=w5820) -> (x*y=w5819:dbl)
                          }
                        }
                        n3192 = local read "SIG LAB01-2"() -> (w5810:T2)
                        n3193 = local read "SIG LAB01-1"() -> (w5812:T2)
                        n3194 = Bundle By Name(cluster=w5812, "Tmp Live"=w5794, "Tmp Neut"=w5792) -> (w5811:T2)
                        n3195 = Bundle By Name(cluster=w5810, "Tmp Live"=w5788, "Tmp Neut"=w5787) -> (w5809:T2)
                        n3196 = local write "SIG LAB01-1"(w5811) -> ()
                        n3197 = local write "SIG LAB01-2"(w5809) -> ()
                      }
                      frame #2 {
                        n3198 = case shown="True" w5842 {
                          tunnel: [w5873 w5874] -> w5858
                          tunnel: w5841 -> [_ w5874]
                          frame False {
                            n3199 = local read "CAL LAB02"() -> (w5873:T15)
                          }
                          frame True {
                          }
                        }
                        n3200 = local read "LAB02 TEMP"() -> (w5849:T12)
                        n3201 = local read "TEMP LA02"() -> (w5848:T9)
                        n3202 = call "sub vi - temperature delay v4.vi"("2-run"=w5830, "1-run"=w5831, "temp values IN"=w5848, "temp signals"=w5849) -> ("T2-N"=w5843:dbl, "T2-L"=w5844:dbl, "T1-N"=w5845:dbl, "T1-L"=w5846:dbl, "temp values OUT"=w5847:T44)  [unwired: 3 in]
                        n3203 = Unbundle By Name(w5858) -> ("1 (TL) cal"=w5853:dbl, "1 (TN) cal"=w5852:dbl, "2 (TL) cal"=w5851:dbl, "2 (TN) cal"=w5850:dbl)  [unwired: 6 out]
                        n3204 = local write "TEMP LA02"(w5847) -> ()
                        n3205 = Multiply(x=w5846, y=w5853) -> (x*y=w5839:dbl)
                        n3206 = Multiply(x=w5845, y=w5852) -> (x*y=w5838:dbl)
                        n3207 = Multiply(x=w5844, y=w5851) -> (x*y=w5835:dbl)
                        n3208 = Multiply(x=w5843, y=w5850) -> (x*y=w5834:dbl)
                        n3209 = case shown="True" w5831 {
                          tunnel: w5839 -> [w5867 w5872]
                          tunnel: w5840 -> [_ w5870]
                          tunnel: [w5867 w5871] -> w5837
                          tunnel: w5838 -> [w5866 w5869]
                          tunnel: [w5866 w5868] -> w5836
                          frame False {
                          }
                          frame True {
                            n3210 = Multiply(x=w5870, y=w5869) -> (x*y=w5868:dbl)
                            n3211 = Multiply(x=w5870, y=w5872) -> (x*y=w5871:dbl)
                          }
                        }
                        n3212 = case shown="True" w5830 {
                          tunnel: w5835 -> [w5860 w5865]
                          tunnel: w5840 -> [_ w5863]
                          tunnel: [w5860 w5864] -> w5833
                          tunnel: w5834 -> [w5859 w5862]
                          tunnel: [w5859 w5861] -> w5832
                          frame False {
                          }
                          frame True {
                            n3213 = Multiply(x=w5863, y=w5862) -> (x*y=w5861:dbl)
                            n3214 = Multiply(x=w5863, y=w5865) -> (x*y=w5864:dbl)
                          }
                        }
                        n3215 = local read "SIG LAB02-2"() -> (w5855:T2)
                        n3216 = local read "SIG LAB02-1"() -> (w5857:T2)
                        n3217 = Bundle By Name(cluster=w5857, "Tmp Live"=w5837, "Tmp Neut"=w5836) -> (w5856:T2)
                        n3218 = Bundle By Name(cluster=w5855, "Tmp Live"=w5833, "Tmp Neut"=w5832) -> (w5854:T2)
                        n3219 = local write "SIG LAB02-1"(w5856) -> ()
                        n3220 = local write "SIG LAB02-2"(w5854) -> ()
                      }
                      frame #3 {
                        n3221 = case shown="False" w5887 {
                          tunnel: [w5918 w5919] -> w5903
                          tunnel: w5886 -> [_ w5919]
                          frame False {
                            n3222 = local read "CAL LAB03"() -> (w5918:T14)
                          }
                          frame True {
                          }
                        }
                        n3223 = local read "TEMP LA03"() -> (w5893:T9)
                        n3224 = local read "LAB03 TEMP"() -> (w5894:T12)
                        n3225 = call "sub vi - temperature delay v4.vi"("2-run"=w5875, "1-run"=w5876, "temp values IN"=w5893, "temp signals"=w5894) -> ("T2-N"=w5888:dbl, "T2-L"=w5889:dbl, "T1-N"=w5890:dbl, "T1-L"=w5891:dbl, "temp values OUT"=w5892:T44)  [unwired: 3 in]
                        n3226 = Unbundle By Name(w5903) -> ("1 (TL) cal"=w5898:dbl, "1 (TN) cal"=w5897:dbl, "2 (TL) cal"=w5896:dbl, "2 (TN) cal"=w5895:dbl)  [unwired: 6 out]
                        n3227 = local write "TEMP LA03"(w5892) -> ()
                        n3228 = Multiply(x=w5891, y=w5898) -> (x*y=w5884:dbl)
                        n3229 = Multiply(x=w5890, y=w5897) -> (x*y=w5883:dbl)
                        n3230 = Multiply(x=w5889, y=w5896) -> (x*y=w5880:dbl)
                        n3231 = Multiply(x=w5888, y=w5895) -> (x*y=w5879:dbl)
                        n3232 = case shown="True" w5875 {
                          tunnel: w5880 -> [w5905 w5910]
                          tunnel: w5885 -> [_ w5908]
                          tunnel: [w5905 w5909] -> w5878
                          tunnel: w5879 -> [w5904 w5907]
                          tunnel: [w5904 w5906] -> w5877
